vi "ErrorTolerance.vi"(7 "Enable":bool, 10 "error tol":dbl, 11 "input":dbl) -> (3 "output":dbl)   [LabVIEW 2019]
panel:
  in  "last input":dbl
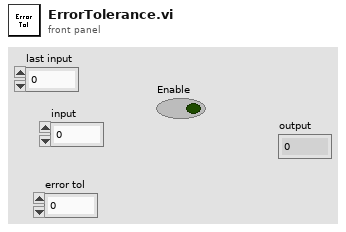
[diagram p1: front panel]
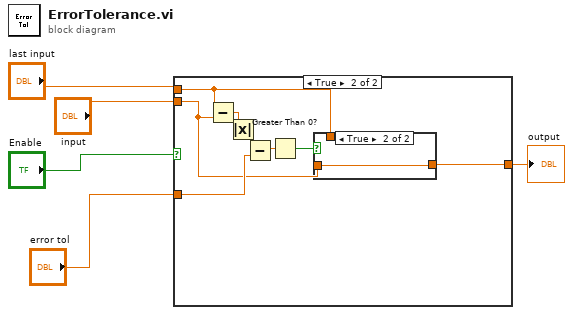
[diagram p0: block diagram]
diagram:
  n1 = case shown="True" "Enable" {
    tunnel: "input" -> [w6 w8]
    tunnel: [w6 w12] -> w4
    tunnel: "error tol" -> [_ w10]
    tunnel: "last input" -> [_ w7]
    frame False {
    }
    frame True {
      n2 = Subtract(x=w7, y=w8) -> (x-y=w9:dbl)
      n3 = Absolute Value(x=w9) -> (abs(x)=w13:dbl)
      n4 = Subtract(x=w13, y=w10) -> (x-y=w14:dbl)
      n5 = Greater Than 0?(x=w14) -> (x > 0?=w11:bool)
      n6 = case shown="True" w11 {
        tunnel: [w15 w16] -> w12
        tunnel: w8 -> [_ w16]
        tunnel: w7 -> [w15 _]
        frame False {
        }
        frame True {
        }
      }
    }
  }
  "output" <- w4
